vi "fgv_F9P_q.vi"(7 "cmd":enum16{"create", "write", "read", "close"}(ring), 8 "error in":errorcluster, 11 "data":enum16{"run", "check", "stop"}(ring)=enum."check") -> (0 "error out":errorcluster, 3 "queue out":refnum<queue>)   [LabVIEW 2019]
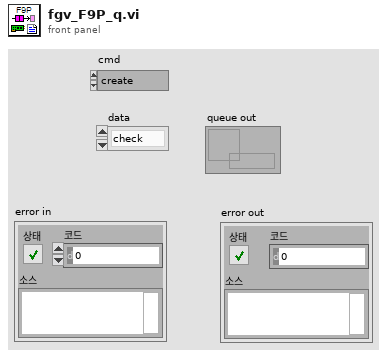
[diagram p1: front panel]
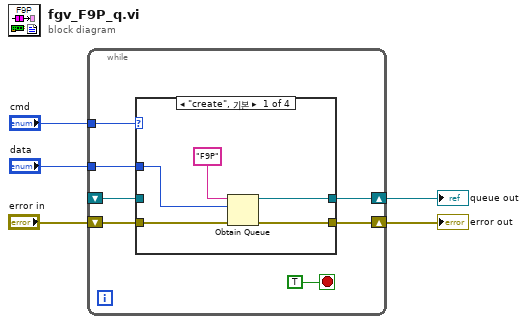
[diagram p0: block diagram]
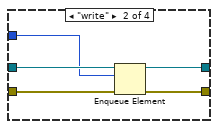
[diagram p2: hidden frame]
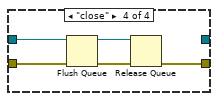
[diagram p4: hidden frame]
diagram:
  n1 = while {
    tunnel: "cmd" -> [w11]
    shift-right: [w9] -> w4
    shift-left: "error in" -> [w10]
    shift-right: [w8] -> w1
    shift-left: _ -> [w7]
    tunnel: "data" -> [w6]
    stop <- TRUE stop-if-true
    n2 = case shown="\"create\", 기본" w11 {
      tunnel: w10 -> [w17 w22 w24 w25]
      tunnel: [w16 w21 w24 w28] -> w9
      tunnel: [w15 w19 w23 _] -> w8
      tunnel: w7 -> [_ w20 w23 w26]
      tunnel: w6 -> [w13 w18 _ _]
      frame "create", Default {
        n3 = Obtain Queue(name (unnamed)="F9P" ("이름(이름없음)"), element data type=w13, error in (no error)=w17) -> (queue out=w15:refnum<queue>, error out=w16:errorcluster)  [unwired: 2 in, 1 out]
      }
      frame "write" {
        n4 = Enqueue Element(queue=w20, element=w18, error in (no error)=w22) -> (queue out=w19:refnum<queue>, error out=w21:errorcluster)  [unwired: 1 in, 1 out]
      }
      frame "read" {
      }
      frame "close" {
        n5 = Flush Queue(queue=w26, error in (no error)=w25) -> (queue out=w27:refnum<queue>, error out=w29:errorcluster)  [unwired: 1 out]
        n6 = Release Queue(queue=w27, error in (no error)=w29) -> (error out=w28:errorcluster)  [unwired: 1 in, 2 out]
      }
    }
  }
  "error out" <- w4
  "queue out" <- w1
